vi "FGV-BroadcastRegistry(lvlibp).vi"(0 "Source":string, 5 "Target":string, 7 "Status":string, 9 "API":string, 11 "Error In":errorcluster caption="error in (no error)", 12 "Operation":T3) -> (4 "Response Message":string[](array[string]), 6 "Values":T1[](array[typedef]), 15 "error out":errorcluster)   [LabVIEW 2017, in "Communicable State Machine.lvlib"]
uses:
  Communicable State Machine.lvlib
  Operation-BroadcastRegistry.ctl
  BroadcastRegistry/BroadcastRegistry-Value.ctl
  AdvanceAPI/CSM - Broadcast Message Type.ctl
  FGV-BroadcastRegistry.vi
  _Shared/CSM Shared.lvlib
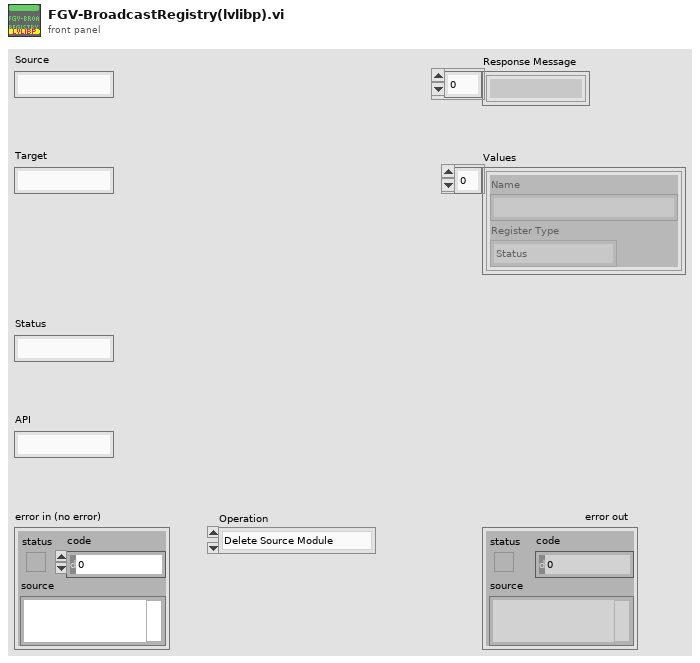
[diagram p1: front panel]
types:
  T1 = typedef "Communicable State Machine.lvlib/BroadcastRegistry-Value.ctl" = cluster{"Name":string, "Register Type":T2}
  T2 = typedef "Communicable State Machine.lvlib/CSM - Broadcast Message Type.ctl" = enum16{"<Null>", "Status", "Interrupt"}
  T3 = typedef "Communicable State Machine.lvlib/Operation-BroadcastRegistry.ctl" = enum16{"Delete Source Module", "Delete Target Module", "Remove Module", "Register", "Unregister", "Check", "List Status", "List Entries", "List Status Of Source", "Drop", "Register As Status", "Register As Interrupt"}
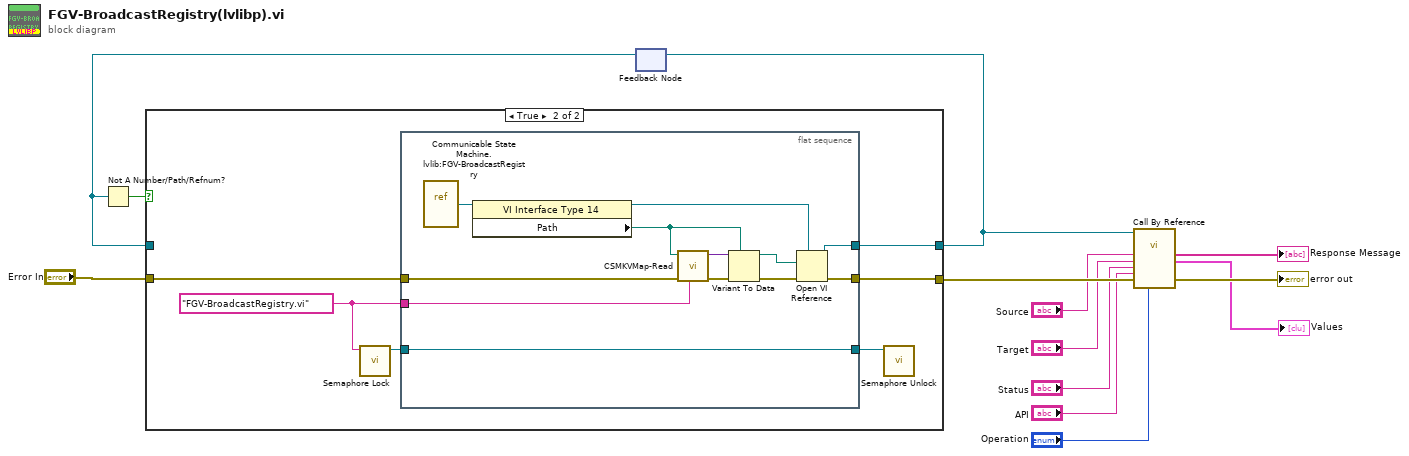
[diagram p0: block diagram]
diagram:
  n1 = feedback #1() -> (w12:refnum<vi>)  [unwired: 1 in]
  n2 = Not A Number/Path/Refnum?(number/path/refnum=w12) -> (NaN/Path/Refnum?=w13:bool)
  n3 = case shown="True" w13 {
    tunnel: [w15 w20] -> w11
    tunnel: w12 -> [w15 _]
    tunnel: [w14 w21] -> w10
    tunnel: "Error In" -> [w14 w19]
    frame False {
    }
    frame True {
      w16 = "FGV-BroadcastRegistry.vi" ("name")
      n4 = call "Semaphore Lock.vi"("name"=w16) -> ("semaphore"=w17:refnum<queue>)  [unwired: 10 in]
      n5 = flat-sequence {
        tunnel: [w29] -> w21
        tunnel: [w27] -> w20
        tunnel: w19 -> [w25]
        tunnel: [w23] -> w18
        tunnel: w17 -> [w23]
        tunnel: w16 -> [w22]
        frame #0 {
          n6 = vi-ref "Communicable State Machine.lvlib:FGV-BroadcastRegistry.vi"() -> (w24:refnum<vi>)
          n7 = property class="VI Interface Type 14"(reference=w24) -> (reference out=w26:refnum<vi>, "Path"=w28:path)  [unwired: 1 in, 1 out]
          n8 = call "CSMKVMap-Read.vi"("name"=w22, "Error in"=w25, "default value (empty variant)"=w28) -> ("Error out"=w33:errorcluster, "value"=w32:variant)  [unwired: 5 in]
          n9 = Variant To Data(error in=w33, type=w28, Variant=w32) -> (data=w31:path, error out=w30:errorcluster)
          n10 = Open VI Reference(type specifier VI Refnum (for type only)=w26, vi path=w31, error in (no error)=w30) -> (vi reference=w27:refnum<vi>, error out=w29:errorcluster)  [unwired: 3 in]
        }
      }
      n11 = call "Semaphore Unlock.vi"("semaphore"=w18) -> ()  [unwired: 11 in]
    }
  }
  n12 = feedback-in #1(w11) -> ()
  n13 = call-by-ref "?"(reference=w11, "Source"="Source", "Target"="Target", "Status"="Status", "API"="API", "Error In"=w10, "Operation"="Operation") -> ("Response Message"=→"Response Message":string[], "Values"=→"Values":T1[], "error out"=→"error out":errorcluster)  [unwired: 8 in, 2 out]
